vi "DecodeCommands.vi"(8 "error in":errorcluster, 9 "Array":u8[](array[numeric]) format="%02x") -> (0 "error out":errorcluster, 1 "array w/ subset deleted":u8[](array[numeric]), 3 "Commands":T1)   [LabVIEW 2017]
uses:
  Varint Decoder uint32.vi
panel:
  in  "Commands":T1
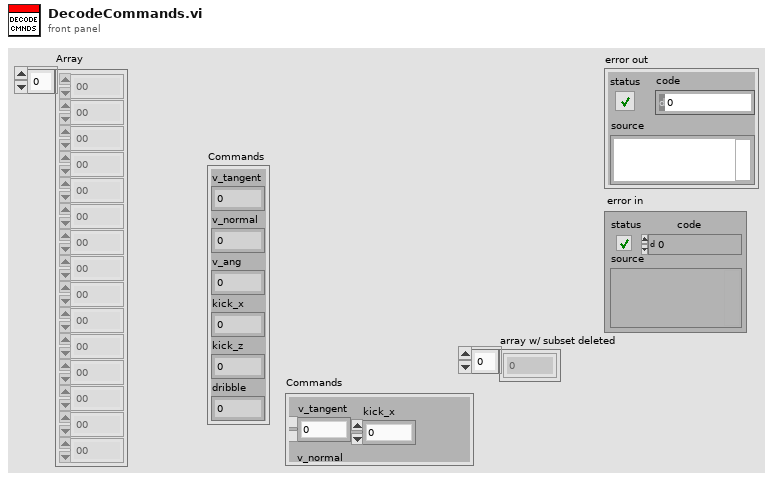
[diagram p1: front panel]
types:
  T1 = cluster{"v_tangent":dbl, "v_normal":dbl, "v_ang":dbl, "kick_x":dbl, "kick_z":dbl, "dribble":u32}
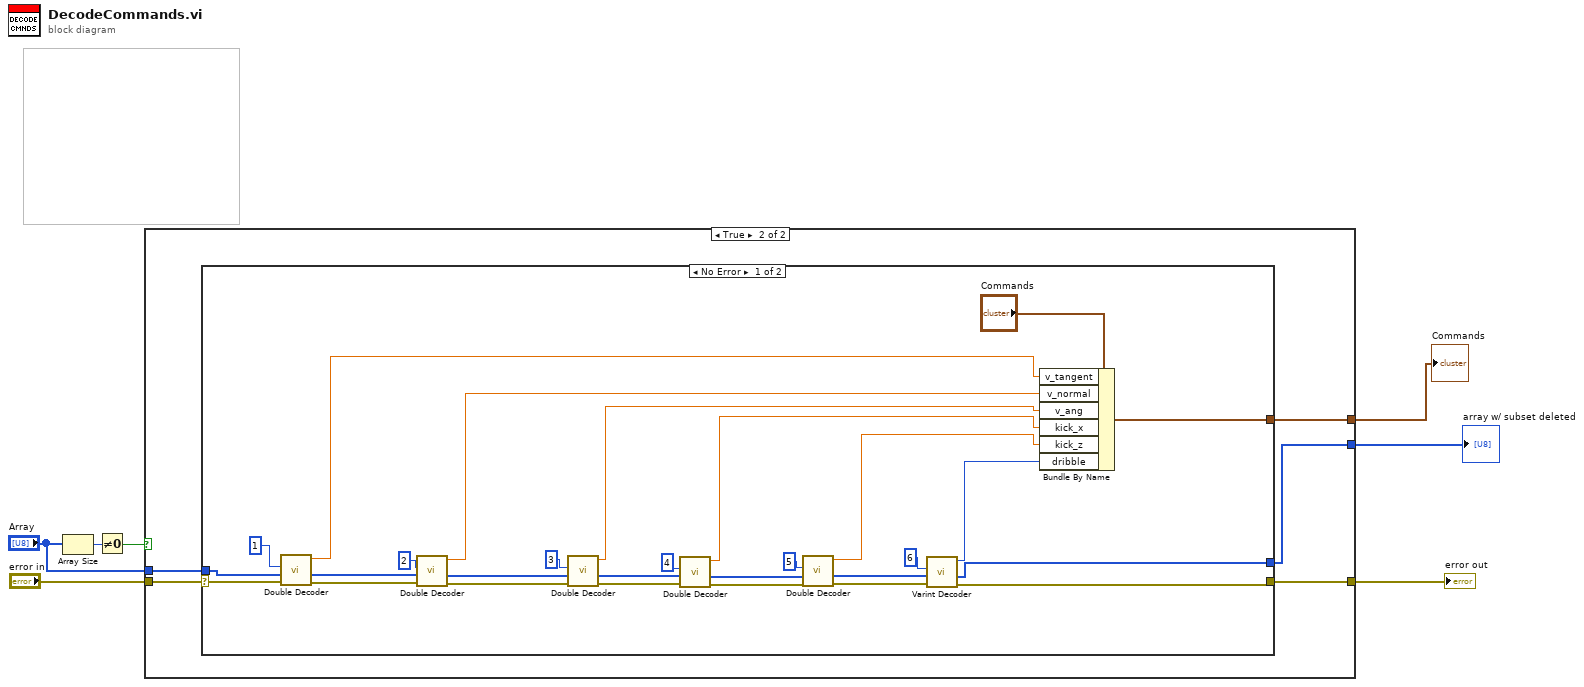
[diagram p0: block diagram]
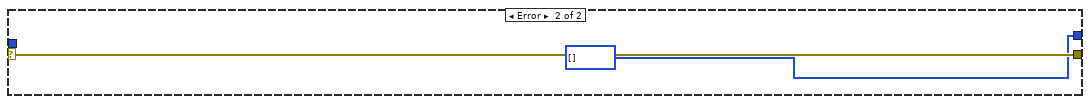
[diagram p3: hidden frame]
diagram:
  n1 = Array Size(array="Array") -> (size(s)=w5:i32)
  n2 = Not Equal To 0?(x=w5) -> (x != 0?=w3:bool)
  n3 = case shown="True" w3 {
    tunnel: "error in" -> [_ w12]
    tunnel: "Array" -> [_ w11]
    tunnel: [_ w10] -> w4
    tunnel: [_ w9] -> w2
    tunnel: [_ w8] -> w1
    frame False {
    }
    frame True {
      n4 = case shown="No Error" w12 {
        selector: w12 -> [w37 w42]
        tunnel: [w22 w42] -> w10
        tunnel: [w23 u8[] [] ("array w/ subset deleted")] -> w9
        tunnel: w11 -> [w38 _]
        tunnel: [w13 _] -> w8
        frame No Error {
          n5 = call "Double Decoder.vi"("error in (no error)"=w37, "Array"=w38, "Key"=1) -> ("error out"=w35:errorcluster, "array w/ subset deleted"=w36:u8[], "Double"=w19:dbl)  [unwired: 5 in, 1 out]
          n6 = call "Double Decoder.vi"("error in (no error)"=w35, "Array"=w36, "Key"=2) -> ("error out"=w40:errorcluster, "array w/ subset deleted"=w39:u8[], "Double"=w18:dbl)  [unwired: 5 in, 1 out]
          n7 = call "Double Decoder.vi"("error in (no error)"=w40, "Array"=w39, "Key"=3) -> ("error out"=w33:errorcluster, "array w/ subset deleted"=w34:u8[], "Double"=w17:dbl)  [unwired: 5 in, 1 out]
          n8 = call "Double Decoder.vi"("error in (no error)"=w33, "Array"=w34, "Key"=4) -> ("error out"=w31:errorcluster, "array w/ subset deleted"=w32:u8[], "Double"=w16:dbl)  [unwired: 5 in, 1 out]
          n9 = call "Double Decoder.vi"("error in (no error)"=w31, "Array"=w32, "Key"=5) -> ("error out"=w24:errorcluster, "array w/ subset deleted"=w25:u8[], "Double"=w15:dbl)  [unwired: 5 in, 1 out]
          n10 = call-poly "Varint Decoder.vi"("error in (no error)"=w24, "Array"=w25, "Key"=6) -> ("error out"=w22:errorcluster, "array w/ subset deleted"=w23:u8[], "Varint"=w14:u32)  [unwired: 5 in, 1 out]
          n11 = Bundle By Name(cluster="Commands", "v_tangent"=w19, "v_normal"=w18, "v_ang"=w17, "kick_x"=w16, "kick_z"=w15, "dribble"=w14) -> (w13:T1)
        }
        frame Error {
        }
      }
    }
  }
  "error out" <- w4
  "array w/ subset deleted" <- w2
  "Commands" <- w1
